vi "Heat Equation Solver(CuLab).vi"() -> ()   [LabVIEW 2020]
doc: "Solves the heat equation in a two-dimensional area using a Finite Element Method."
uses:
  <vilib>/Utility/miscctls.llb/LVPointDoubleTypeDef.ctl
  <vilib>/picture/3D Picture Control/Object/Create Object (name).vi
  <vilib>/Ngene/CuLab - GPU Accelerated Toolkit/Toolkit/Low_Level/Tensor_Classes/T_Children/T2D/T2D_Children/T2D_SGL/Create_Push.vi
  <vilib>/Ngene/CuLab - GPU Accelerated Toolkit/Toolkit/API/Array/Initialize Array/T1D/CU_Initialize Array_T1D_SGL.vi
  <vilib>/Ngene/CuLab - GPU Accelerated Toolkit/Toolkit/Low_Level/Tensor_Classes/T_Children/T1D/T1D_Children/T1D_SGL/Push.vi
  <vilib>/Ngene/CuLab - GPU Accelerated Toolkit/Toolkit/API/Linear Algebra/BLAS2/gemv/CU_gemv/CU_Sgemv.vi
  <vilib>/Ngene/CuLab - GPU Accelerated Toolkit/Toolkit/API/Numeric/Add/T1D/CU_Add_T1D_SGL.vi
  <vilib>/Ngene/CuLab - GPU Accelerated Toolkit/Toolkit/API/Linear Algebra/BLAS1/axpy/CU_axpy/CU_Saxpy.vi
  <vilib>/Ngene/CuLab - GPU Accelerated Toolkit/Toolkit/Low_Level/Tensor_Classes/T_Children/T1D/T1D_Children/T1D_SGL/Pull.vi
  subVIs/Heat Equation Solver.lvlib
  <vilib>/picture/3D Picture Control/NI_3D Picture Control.lvlib
  <vilib>/Ngene/CuLab - GPU Accelerated Toolkit/Toolkit/CuLab.lvlib
  <vilib>/ptbypt/NI_PtbyPt.lvlib
  <vilib>/Ngene/CuLab - GPU Accelerated Toolkit/Toolkit/Low_Level/Tensor_Classes/T_Children/T2D/T2D_Children/T2D_SGL/T2D_SGL.lvclass
  <vilib>/Ngene/CuLab - GPU Accelerated Toolkit/Toolkit/Low_Level/Tensor_Classes/T_Children/T1D/T1D_Children/T1D_SGL/T1D_SGL.lvclass
panel:
  out "stop display":bool
  out "Heat Map":sgl[](array[numeric])
  out "sol":refnum<vi>(3d-picture) caption="Heat Distribution"
  out "colorbar":sgl[][](graph)
  out "time":dbl[unit] format="%#_4p"
  out "time graph":dbl(graph)
  out "Error out":errorcluster
  in  "radius":dbl(slide)=0.15 caption="Radius" min=0.1 max=0.3 step=0.01 scale=0.1..0.2
  out "tri":cluster{"X":dbl[], "Y":dbl[]}[](graph) caption="Triangulation"
  in  "stop":bool
  # "Heat Equation Solver based on CuLab"
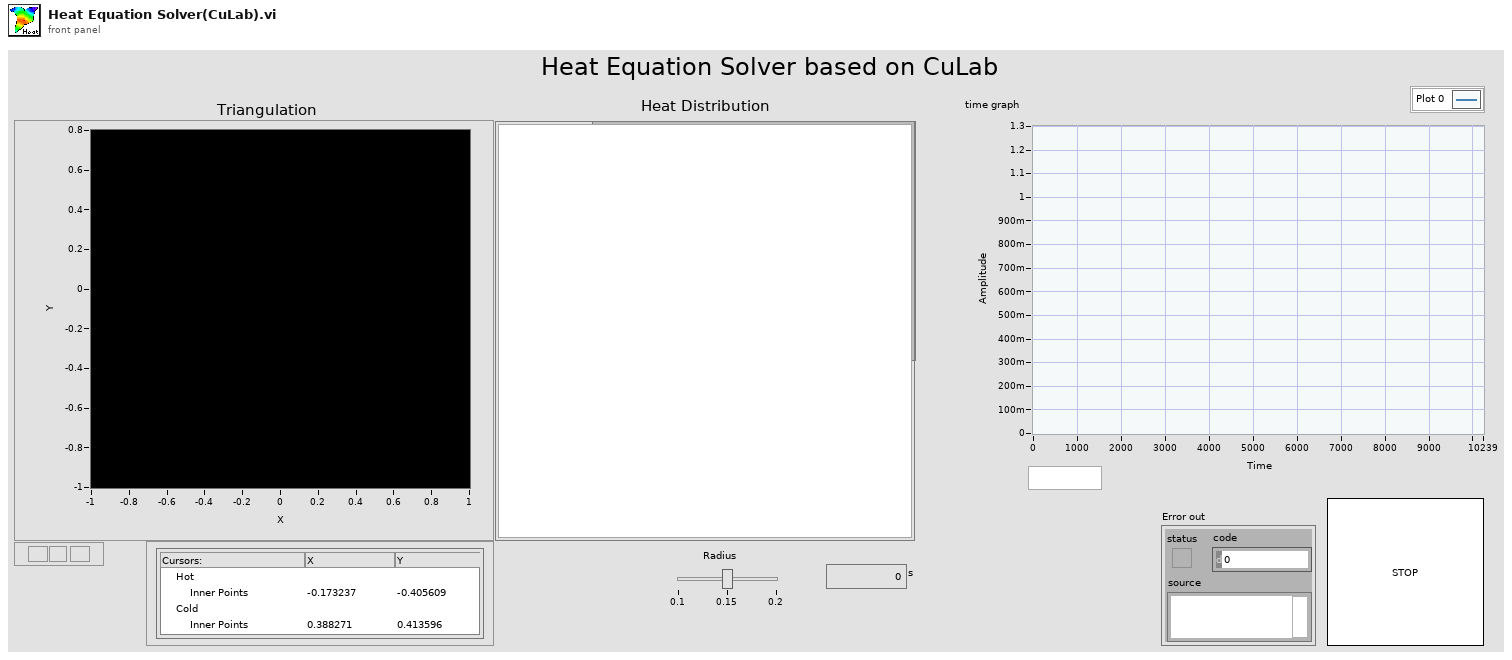
[diagram p1: front panel]
types:
  T1 = typedef "Heat Equation Solver.lvlib/FEM Grid.ctl" = cluster{"X":dbl[], "Y":dbl[], "Trianglation":i32[][]}
  T2 = typedef "NI_Matrix.lvlib/RealMatrix.ctl" = dbl[][]
  T3 = typedef "LVPointDoubleTypeDef.ctl" = cluster{"X":dbl, "Y":dbl}
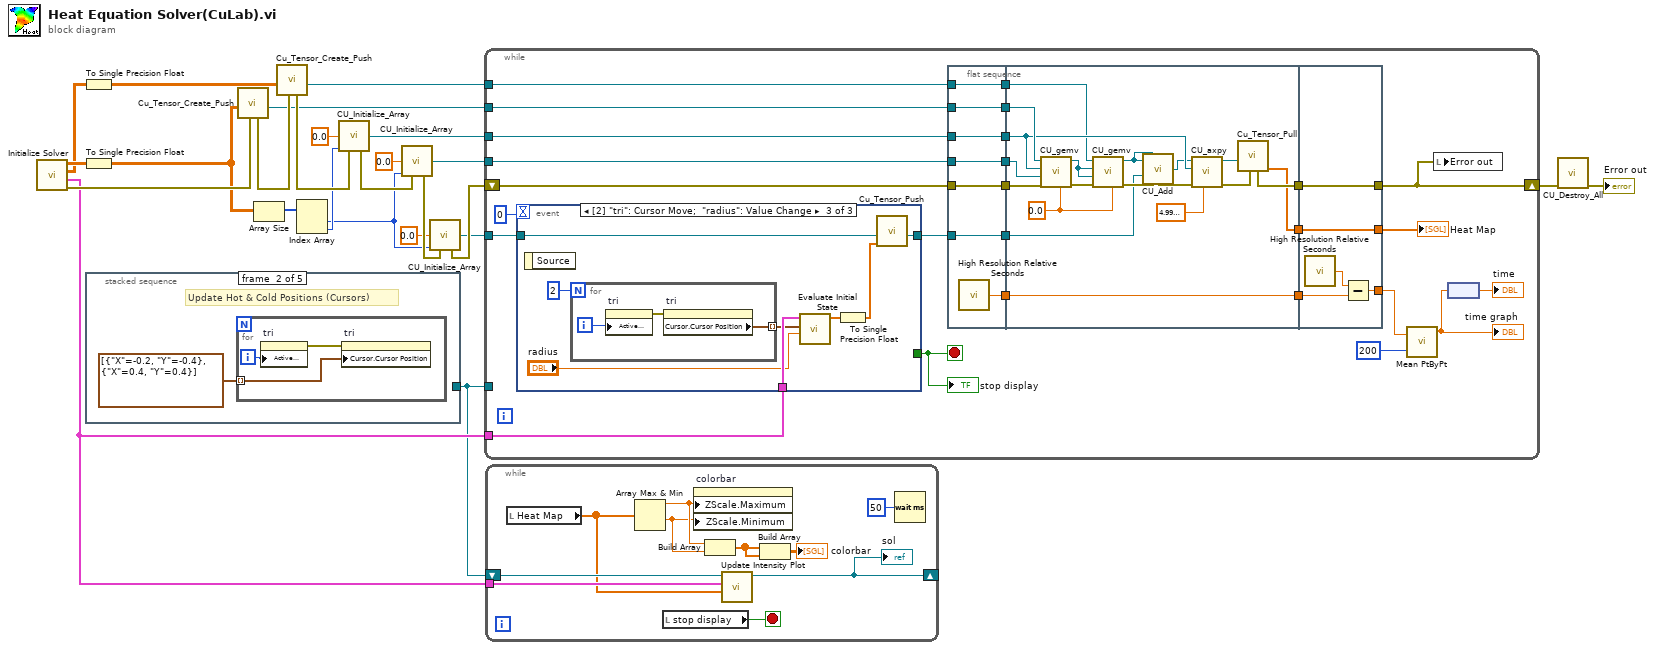
[diagram p0: block diagram]
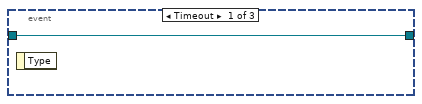
[diagram p2: hidden frame]
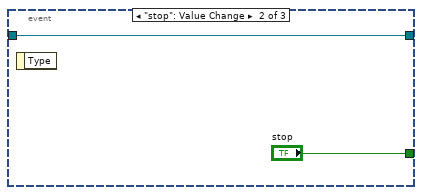
[diagram p3: hidden frame]
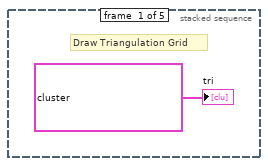
[diagram p4: hidden frame]
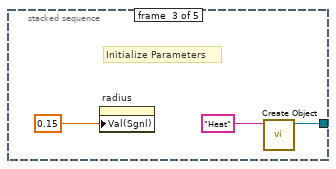
[diagram p5: hidden frame]
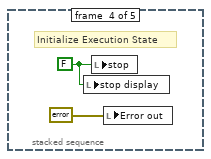
[diagram p6: hidden frame]
diagram:
  n1 = call "Initialize Solver.vi"() -> ("error out"=w23:errorcluster, "FEM Grid"=w3:T1, "Mass"=w13:T2, "Stiffness"=w17:T2)  [unwired: 8 in]
  n2 = To Single Precision Float(number=w13) -> (single precision float=w11:sgl[][])
  n3 = To Single Precision Float(number=w17) -> (single precision float=w12:sgl[][])
  n4 = stacked-sequence {
    tunnel: [_ _ w32 _ _] -> w2
    frame #0 {
      # "Draw Triangulation Grid"
      "tri" <- cluster{"X":dbl[], "Y":dbl[]}[] [{"X"=array[689 elements], "Y"=array[689 elements]}, {"X"=[-0.825, -0.8029029130879204, -0.8, -0.775, -0.7625, -0.7375, -0.725, -0.7, -0.6875, -0.6625, -0.65, -0.625, -0.6125, -0.5875, -0.575, -0.55, -0.5375, -0.5125, -0.5, -0.475, -0.4625, -0.44999999999999996, -0.44999999999999996, -0.44999999999999996, -0.44999999999999996, -0.44999999999999996, -0.44375, -0.44375, -0.44375, -0.4375, -0.4375, -0.43125, -0.43125, -0.42500000000000004, -0.42500000000000004, -0.42500000000000004, -0.41250000000000003, -0.4125, -0.4, -0.3875, -0.3875, -0.38125, -0.375, -0.375, -0.36875, -0.36250000000000004, -0.35625, -0.35, -0.35, -0.35, -0.34375, -0.34375, -0.3375, -0.3375, -0.3375, -0.33749999999999997, -0.33125, -0.32499999999999996, -0.32499999999999996, -0.32499999999999996, -0.3125, -0.3125, -0.2875, -0.275, -0.26249999999999996, -0.2375, -0.23124999999999996, -0.19999999999999996, -0.19999999999999996, -0.16874999999999996, -0.16249999999999998, -0.13749999999999996, -0.125, -0.09999999999999998, -0.08750000000000002, -0.0625, -0.050000000000000044, -0.025000000000000022, -0.012500000000000067, 0.012499999999999956, 0.02499999999999991, 0.025000000000000022, 0.03750000000000009, 0.03750000000000009, 0.03750000000000009, 0.03750000000000009, 0.03750000000000009, 0.0625, 0.10000000000000009, 0.10000000000000009, 0.13750000000000007, 0.13750000000000007, 0.17500000000000004, 0.17500000000000004, 0.19374999999999998, 0.2124999999999999, 0.21250000000000002, 0.2437499999999999, 0.25, 0.2749999999999999, 0.2875, 0.32499999999999996, 0.3374999999999999, 0.36249999999999993, 0.375, 0.3999999999999999, 0.4125000000000001, 0.4375, 0.45000000000000007, 0.4750000000000001, 0.48750000000000004, 0.5125000000000001, 0.525, 0.55, 0.5625, 0.5875, 0.6, 0.625, 0.6375, 0.65625, 0.6625000000000001, 0.6625000000000001, 0.6625000000000001, 0.6687500000000001, 0.6749999999999999, 0.675, 0.675, 0.675, 0.675, 0.68125, 0.6875, 0.6875, 0.7, 0.7124999999999999, 0.7124999999999999, 0.725, 0.7375, 0.75, 0.7625000000000001, 0.7875000000000001, 0.7875000000000001, 0.80625, 0.825, 0.8250000000000001, 0.85625, 0.8625, 0.8875, 0.9, 0.90625, 0.9249999999999999, 0.9375, 0.9624999999999999], "Y"=[0.575, 0.5529029130879203, 0.6000000000000001, 0.5249999999999999, 0.61875, 0.5125, 0.6375, 0.5, 0.65625, 0.475, 0.675, 0.44999999999999996, 0.69375, 0.42499999999999993, 0.7124999999999999, 0.3999999999999999, 0.71875, 0.36249999999999993, 0.7250000000000001, 0.32499999999999996, 0.7312500000000001, -0.7875, -0.75, -0.7125, -0.675, -0.6375, -0.825, -0.6, 0.2875, -0.8625, -0.5625, -0.9, -0.525, -0.9375, -0.48750000000000004, 0.7375, -0.45, 0.25, -0.4125, -0.375, 0.74375, 0.21875, -0.925, -0.3375, -0.3, -0.26249999999999996, -0.22499999999999998, -0.1875, 0.1875, 0.75, -0.8875, -0.15000000000000002, -0.11250000000000004, -0.07500000000000001, -0.03749999999999998, 0.15000000000000002, 5.551115123125783e-17, 0.03750000000000009, 0.07500000000000007, 0.11250000000000004, -0.85, 0.75, -0.8125, 0.75, -0.775, 0.75, -0.74375, -0.7125, 0.75, -0.68125, 0.74375, -0.65, 0.7375, -0.61875, 0.71875, -0.5875, 0.7, -0.55625, 0.6749999999999999, -0.525, 0.6499999999999999, -0.4875, -0.44999999999999996, -0.4125, -0.375, -0.3375, -0.30000000000000004, 0.6124999999999999, -0.32499999999999996, 0.575, -0.35, 0.54375, -0.375, 0.5125, 0.5499999999999999, 0.5874999999999999, -0.36875, 0.625, -0.36250000000000004, 0.6625000000000001, -0.35000000000000003, -0.3375, 0.7, -0.31875000000000003, 0.7062499999999999, -0.30000000000000004, 0.7124999999999999, -0.28125, 0.725, -0.26249999999999996, 0.7375, -0.24374999999999997, 0.7375, -0.22499999999999998, 0.7375, -0.20625, 0.74375, -0.1875, 0.75, -0.16249999999999998, 0.08749999999999991, 0.13124999999999998, 0.17500000000000004, 0.04999999999999993, 0.75, -0.0625, -0.025000000000000022, 0.012499999999999956, 0.21250000000000002, -0.09999999999999998, -0.13749999999999996, 0.25, 0.2875, 0.32499999999999996, 0.75, 0.36249999999999993, 0.3999999999999999, 0.75, 0.4375, 0.4750000000000001, 0.75, 0.5125000000000001, 0.55, 0.75, 0.5875, 0.75, 0.625, 0.75, 0.64375, 0.6625, 0.75, 0.7]}, {"X"=array[456 elements], "Y"=array[456 elements]}, {"X"=array[7640 elements], "Y"=array[7640 elements]}] ("Triangulation Plot")
    }
    frame #1 {
      # "Update Hot & Cold Positions (Cursors)"
      n5 = for {
        tunnel: T3[] [{"X"=-0.2, "Y"=-0.4}, {"X"=0.4, "Y"=0.4}] -> [w29] mode=indexing
        i -> [w30]
        n6 = property on="tri" class="XYGraph (strict)"("Active Cursor"=w30) -> (error out=w28:errorcluster)  [unwired: 2 in, 1 out]
        n7 = property on="tri" class="XYGraph (strict)"(error in=w28, "Cursor.Cursor Position"=w29) -> ()  [unwired: 1 in, 2 out]
      }
    }
    frame #2 {
      # "Initialize Parameters"
      n8 = property on="radius" class="Slide (strict)"("Val(Sgnl)"=0.15 ("r")) -> ()  [unwired: 2 in, 2 out]
      n9 = call-poly <vilib>:"Create Object.vi"("Name"="Heat") -> ("Scene:New Object"=w32:refnum<vi>)  [unwired: 9 in, 1 out]
    }
    frame #3 {
      w34 = FALSE ("stop")
      # "Initialize Execution State"
      n10 = local write "stop display"(w34) -> ()
      n11 = local write "stop"(w34) -> ()
      n12 = local write "Error out"(errorcluster {"status"=FALSE, "code"=0, "source"=""} ("Error Status")) -> ()
    }
    frame #4 {
      # "Initialize GPU Information"
    }
  }
  n13 = call-poly <vilib>:"Cu_Tensor_Create_Push.vi"("error in (no error)"=w23, "CPU_Data_2D_SGL"=w12) -> ("T2D_SGL out"=w19:refnum<class "T2D_SGL.lvclass">, "error out"=w22:errorcluster)  [unwired: 8 in]
  n14 = Array Size(array=w12) -> (size(s)=w16:i32[])
  n15 = call-poly <vilib>:"Cu_Tensor_Create_Push.vi"("error in (no error)"=w22, "CPU_Data_2D_SGL"=w11) -> ("T2D_SGL out"=w18:refnum<class "T2D_SGL.lvclass">, "error out"=w21:errorcluster)  [unwired: 8 in]
  n16 = Index Array(array=w16) -> (element #1=w4:i32, element #2=w14:i32)  [unwired: 2 in]
  n17 = call-poly <vilib>:"CU_Initialize_Array.vi"("element"=sgl 0.0 ("SGL"), "dimension size"=w14, "error in (no error)"=w21) -> ("initialized Tensor"=w15:refnum<class "T1D_SGL.lvclass">, "error out"=w9:errorcluster)  [unwired: 11 in]
  n18 = call-poly <vilib>:"CU_Initialize_Array.vi"("element"=sgl 0.0 ("SGL"), "dimension size"=w4, "error in (no error)"=w9) -> ("initialized Tensor"=w10:refnum<class "T1D_SGL.lvclass">, "error out"=w24:errorcluster)  [unwired: 11 in]
  n19 = call-poly <vilib>:"CU_Initialize_Array.vi"("element"=sgl 0.0 ("SGL"), "dimension size"=w4, "error in (no error)"=w24) -> ("initialized Tensor"=w7:refnum<class "T1D_SGL.lvclass">, "error out"=w25:errorcluster)  [unwired: 11 in]
  n20 = while {
    tunnel: w3 -> [w53]
    shift-right: [w47] -> w20
    shift-left: w25 -> [w48]
    tunnel: w18 -> [w55]
    tunnel: w19 -> [w54]
    tunnel: w15 -> [w51]
    tunnel: w10 -> [w44]
    tunnel: w7 -> [w37]
    tunnel: w2 -> [_]
    stop <- w57 stop-if-true
    n21 = event shown="[2] \"tri\": Cursor Move;  \"radius\": Value Change" {
      selector: _ -> [_ _ _]
      dyn-events: _ -> [_ _ _]
      timeout: 0 -> [_ _ _]
      tunnel: [w93 w94 w98] -> w46
      tunnel: [_ "stop" _] -> w57
      tunnel: w53 -> [_ _ w102]
      tunnel: w37 -> [w93 w94 w97]
      event Timeout {
        n22 = event-data() -> ()  [unwired: 1 in, 1 out]
      }
      event "stop": Value Change {
        n23 = event-data() -> ()  [unwired: 1 in, 1 out]
      }
      event "tri": Cursor Move; "radius": Value Change {
        n24 = event-data() -> ()  [unwired: 1 in, 1 out]
        n25 = for {
          N: 2 -> [_]
          tunnel: [w104] -> w100 mode=indexing
          i -> [w106]
          n26 = property on="tri" class="XYGraph (strict)"("Active Cursor"=w106) -> (error out=w105:errorcluster)  [unwired: 2 in, 1 out]
          n27 = property on="tri" class="XYGraph (strict)"(error in=w105) -> ("Cursor.Cursor Position"=w104:T3)  [unwired: 1 in, 2 out]
        }
        n28 = call "Evaluate Initial State.vi"("r"="radius", "Heat Source"=w100, "FEM Grid"=w102) -> ("Initial"=w103:dbl[])  [unwired: 8 in]
        n29 = To Single Precision Float(number=w103) -> (single precision float=w96:sgl[])
        n30 = call-poly <vilib>:"Cu_Tensor_Push.vi"("CPU_Data_1D_SGL"=w96, "T1D_SGL in"=w97) -> ("T1D_SGL out"=w98:refnum<class "T1D_SGL.lvclass">)  [unwired: 8 in, 1 out]
      }
    }
    "stop display" <- w57
    n31 = flat-sequence {
      tunnel: w55 -> [w67]
      tunnel: w54 -> [w68]
      tunnel: [w68] -> w61
      tunnel: [w67] -> w60
      tunnel: [w66] -> w59
      tunnel: w46 -> [w65]
      tunnel: [w65] -> w56
      tunnel: [w64] -> w52
      tunnel: w51 -> [w64]
      tunnel: [w63] -> w50
      tunnel: w48 -> [w63]
      tunnel: [w62] -> w45
      tunnel: w44 -> [w62]
      tunnel: w61 -> [w82]
      tunnel: w60 -> [w72]
      tunnel: w59 -> [w84]
      tunnel: [w84] -> w58
      tunnel: w56 -> [w70]
      tunnel: w52 -> [w75]
      tunnel: w50 -> [w83]
      tunnel: [w86] -> w49
      tunnel: w45 -> [w79]
      tunnel: [w80] -> w43
      tunnel: w58 -> [w92]
      tunnel: w49 -> [w90]
      tunnel: [w90] -> w47
      tunnel: [w89] -> w36
      tunnel: w43 -> [w89]
      tunnel: [w88] -> w39
      frame #0 {
        n32 = call <vilib>:"High Resolution Relative Seconds.vi"() -> ("relative seconds"=w66:dbl)
      }
      frame #1 {
        w73 = sgl 0.0 ("beta")
        n33 = call-poly <vilib>:"CU_gemv.vi"("beta"=w73, "error in (no error)"=w83, "y"=w79, "x"=w75, "A"=w82) -> ("error out"=w81:errorcluster, "y out"=w71:refnum<class "T1D_SGL.lvclass">)  [unwired: 5 in]
        n34 = call-poly <vilib>:"CU_gemv.vi"("beta"=w73, "error in (no error)"=w81, "y"=w71, "x"=w71, "A"=w72) -> ("error out"=w85:errorcluster, "y out"=w78:refnum<class "T1D_SGL.lvclass">)  [unwired: 5 in]
        n35 = call-poly <vilib>:"CU_Add.vi"("Dest in"=w78, "x"=w78, "y"=w70, "error in (no error)"=w85) -> ("Dest out"=w69:refnum<class "T1D_SGL.lvclass">, "error out"=w76:errorcluster)  [unwired: 10 in]
        n36 = call-poly <vilib>:"CU_axpy.vi"("alpha"=sgl 5e-05 ("dt"), "error in (no error)"=w76, "y"=w75, "x"=w69) -> ("error out"=w87:errorcluster, "y out"=w74:refnum<class "T1D_SGL.lvclass">)  [unwired: 6 in]
        n37 = call-poly <vilib>:"Cu_Tensor_Pull.vi"("error in (no error)"=w87, "T1D_SGL in"=w74) -> ("Dest out"=w80:sgl[], "error out"=w86:errorcluster)  [unwired: 7 in, 1 out]
      }
      frame #2 {
        n38 = call <vilib>:"High Resolution Relative Seconds.vi"() -> ("relative seconds"=w91:dbl)
        n39 = Subtract(x=w91, y=w92) -> (x-y=w88:dbl)
      }
    }
    n40 = call <vilib>:"Mean PtByPt.vi"("x"=w39, "sample length"=200) -> ("mean"=w40:dbl)  [unwired: 2 in, 1 out]
    "time graph" <- w40
    n41 = local write "Error out"(w47) -> ()
    n42 = node(w40) -> (→"time":dbl[unit])
    "Heat Map" <- w36
  }
  n43 = while {
    tunnel: w3 -> [w115]
    shift-right: [w113] -> _
    shift-left: w2 -> [w116]
    stop <- w114 stop-if-true
    n44 = local read "Heat Map"() -> (w111:sgl[])
    n45 = Array Max & Min(array=w111) -> (max value=w110:sgl, min value=w109:sgl)  [unwired: 2 out]
    n46 = local read "stop display"() -> (w114:bool)
    n47 = property on="colorbar" class="IntGraph (strict)"("ZScale.Maximum"=w110, "ZScale.Minimum"=w109) -> ()  [unwired: 2 in, 2 out]
    n48 = Build Array(w110, w109) -> (w107:sgl[])
    n49 = call "Update Intensity Plot.vi"("Z"=w111, "FEM Grid"=w115, "FEM plot in"=w116) -> ("FEM plot out"=w113:refnum<vi>)  [unwired: 8 in]
    "sol" <- w113
    n50 = Build Array(w107, w107) -> (→"colorbar":sgl[][])
    n51 = Wait (ms)(milliseconds to wait=u32 50) -> ()  [unwired: 1 out]
  }
  n52 = call <vilib>:"CU_Destroy_All.vi"("error in"=w20) -> ("error out"=→"Error out":errorcluster)  [unwired: 10 in]
